vi "openCommunication.vi"(8 "error in (no error)":errorcluster, 11 "cRIO in":refnum<class "cRIO.lvclass">) -> (0 "error out":errorcluster, 3 "cRIO out":refnum<class "cRIO.lvclass">)   [LabVIEW 2020, in "cRIO.lvclass"]
uses:
  cRIO.lvclass
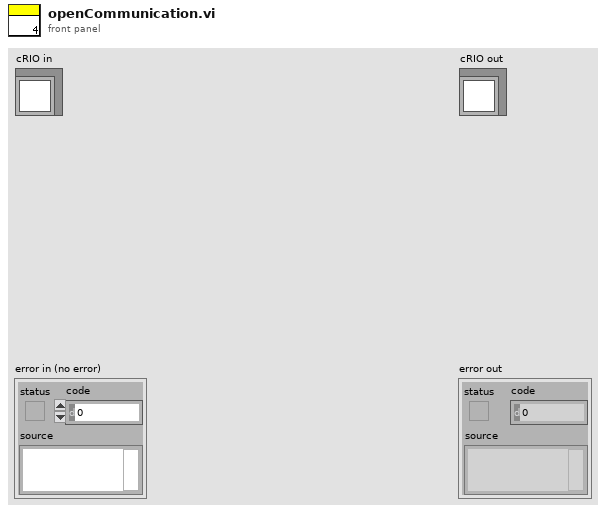
[diagram p1: front panel]
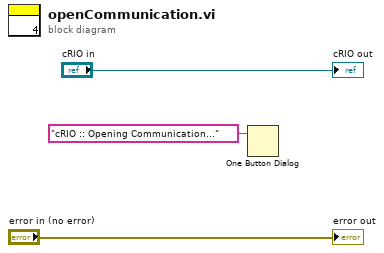
[diagram p0: block diagram]
diagram:
  n1 = One Button Dialog(message="cRIO :: Opening Communication...") -> ()  [unwired: 1 in, 1 out]
  "error out" <- "error in (no error)"
  "cRIO out" <- "cRIO in"
